vi "CreateDatabase.vi"(8 "错误输入（无错误）":errorcluster, 11 "测试类型":string) -> (0 "error out":errorcluster, 3 "数据库地址":string)   [LabVIEW 2014]
uses:
  <vilib>/addons/database/Connection.llb/DB Tools Open Connec (String).vi
  <vilib>/addons/database/Connection.llb/Conn Execute.vi
  <vilib>/addons/database/Recordset.llb/Rec Destroy - Connection.vi
  <vilib>/addons/database/NI_Database_API.lvlib
panel:
  out "error out 2":errorcluster
  out "连接的字符串 2":string
  in  "ADOX._Catalog":refnum<k7>
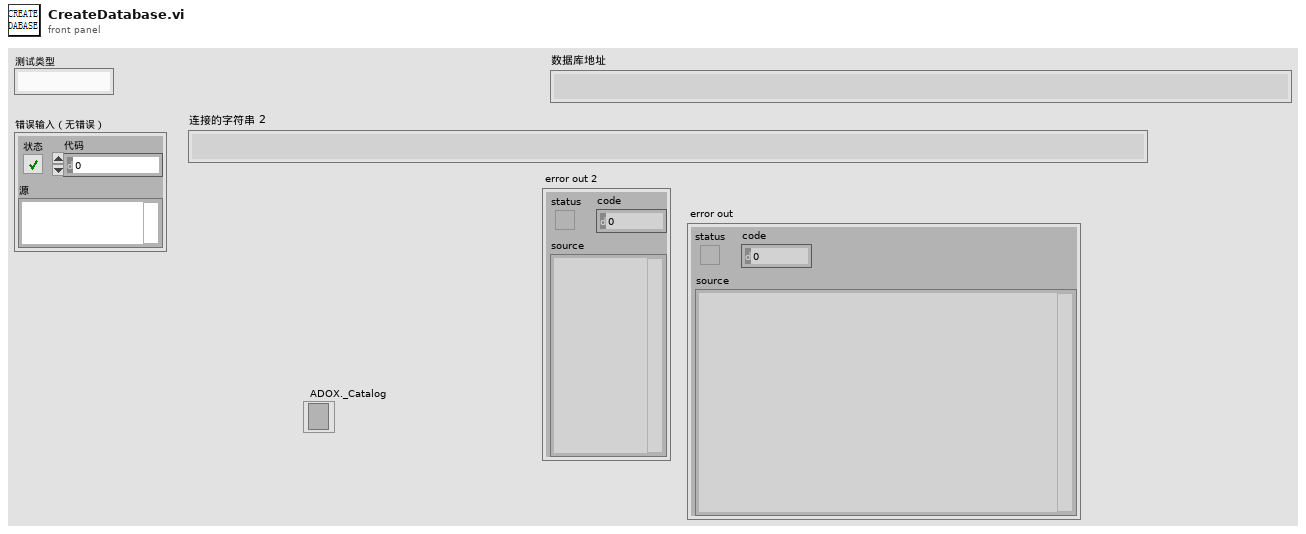
[diagram p1: front panel]
types:
  T1 = typedef "NI_Database_API.lvlib/Conn ObjectReference.ctl" = refnum<k1>
  T2 = typedef "NI_Database_API.lvlib/Rec ObjectReference.ctl" = refnum<k1>
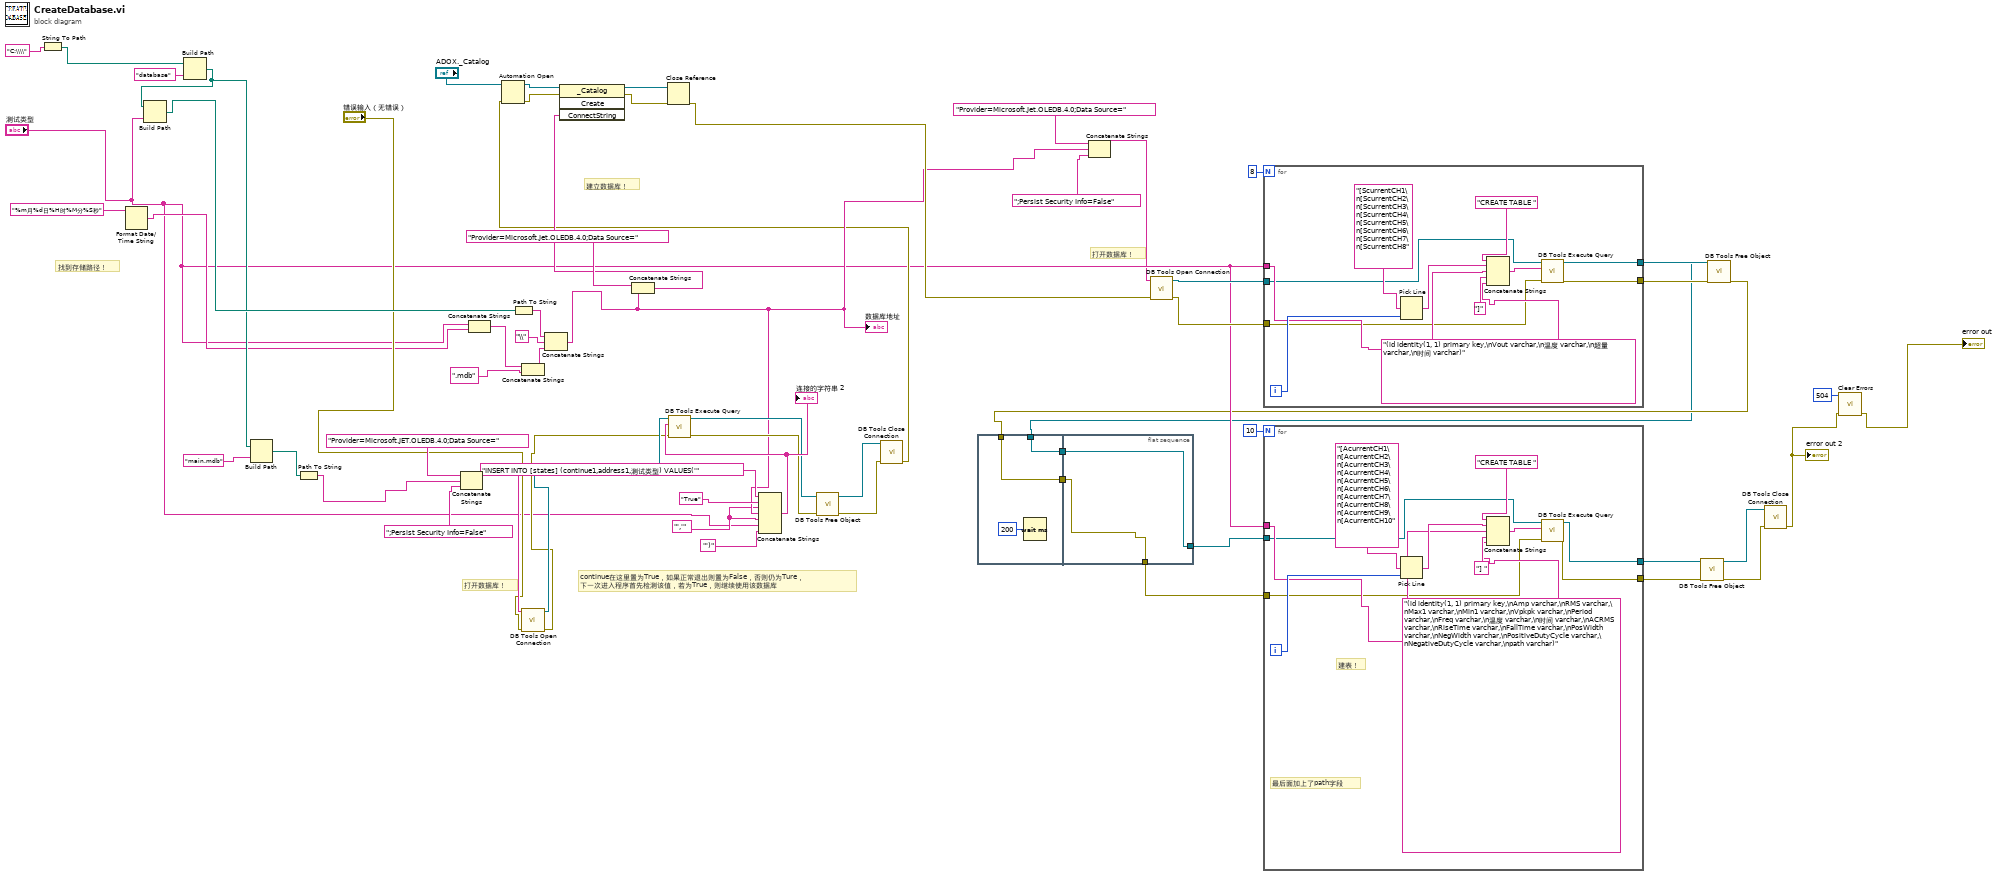
[diagram p0: block diagram]
diagram:
  w17 = "','"
  # "打开数据库！"
  # "continue在这里置为True，如果正常退出则置为False，否则仍为Ture，\n下一次进入程序首先检测该值，若为True，则继续使用该数据库"
  # "打开数据库！"
  # "建立数据库！"
  # "找到存储路径！"
  n1 = String To Path(string="C:\\\\") -> (path=w1:path)
  n2 = Format Date/Time String(time format string (%c)="%m月%d日%H时%M分%S秒" ("时间格式字符串(%c)")) -> (date/time string=w23:string)  [unwired: 2 in]
  n3 = Build Path(base path=w1, name or relative path="database" ("名称或相对路径")) -> (appended path=w34:path)
  n4 = Build Path(base path=w34, name or relative path="测试类型") -> (appended path=w49:path)
  n5 = Build Path(base path=w34, name or relative path="main.mdb" ("名称或相对路径")) -> (appended path=w32:path)
  n6 = Path To String(path=w32) -> (string=w31:string)
  n7 = Concatenate Strings("Provider=Microsoft.JET.OLEDB.4.0;Data Source=", w31, ";Persist Security Info=False") -> (w38:string)
  n8 = Concatenate Strings("测试类型", w23) -> (w20:string)
  n9 = Path To String(path=w49) -> (string=w51:string)
  n10 = Concatenate Strings(w20, ".mdb" ("字符串")) -> (w21:string)
  n11 = call-poly <vilib>:"DB Tools Open Connection.vi"("error in (no error)"="错误输入（无错误）", "connection information"=w38) -> ("error out"=w29:errorcluster, "connection reference"=w30:T1)  [unwired: 6 in]
  n12 = Concatenate Strings(w51, "\\" ("字符串"), w21) -> (w19:string)
  "数据库地址" <- w19
  n13 = Concatenate Strings("Provider=Microsoft.Jet.OLEDB.4.0;Data Source=", w19) -> (w57:string)
  n14 = Concatenate Strings("INSERT INTO [states] (continue1,address1,测试类型) VALUES('", "True", w17, w19, w17, "测试类型", "')") -> (w35:string)
  "连接的字符串 2" <- w35
  n15 = call-poly <vilib>:"DB Tools Execute Query.vi"("error in (no error)"=w29, "SQL query"=w35, "connection reference"=w30) -> ("error out"=w24:errorcluster, "recordset reference"=w25:T2)  [unwired: 5 in]
  n16 = call-poly <vilib>:"DB Tools Free Object.vi"("error in (no error)"=w24, "recordset reference"=w25) -> ("error out"=w26:errorcluster, "connection reference"=w27:T1)  [unwired: 8 in]
  n17 = call <vilib>:"DB Tools Close Connection.vi"("error in (no error)"=w26, "connection reference"=w27) -> ("error out"=w18:errorcluster)  [unwired: 5 in]
  n18 = Automation Open(error in (no error)=w18, Automation Refnum="ADOX._Catalog") -> (Automation Refnum=w62:refnum<k7>, error out=w61:errorcluster)  [unwired: 2 in]
  n19 = invoke class="_Catalog" method="Create"(reference=w62, error in=w61, "ConnectString"=w57) -> (reference out=w60:refnum<k7>, error out=w59:errorcluster)  [unwired: 1 in, 2 out]
  n20 = Close Reference(reference=w60, error in (no error)=w59) -> (error out=w54:errorcluster)
  n21 = flat-sequence {
    tunnel: w8 -> [w65]
    tunnel: [w65] -> w12
    tunnel: w7 -> [w64]
    tunnel: [w64] -> w6
    tunnel: w12 -> [w67]
    tunnel: [w68] -> w10
    tunnel: [w67] -> w9
    tunnel: w6 -> [w68]
    frame #0 {
      n22 = Wait (ms)(milliseconds to wait=u32 200 ("等待时间（毫秒）")) -> ()  [unwired: 1 out]
    }
    frame #1 {
    }
  }
  n23 = Concatenate Strings("Provider=Microsoft.Jet.OLEDB.4.0;Data Source=", w19, ";Persist Security Info=False") -> (w11:string)
  n24 = call-poly <vilib>:"DB Tools Open Connection.vi"("error in (no error)"=w54, "connection information"=w11) -> ("error out"=w41:errorcluster, "connection reference"=w42:T1)  [unwired: 6 in]
  n25 = for {
    N: 8 -> [_]
    tunnel: "测试类型" -> [w75]
    tunnel: w42 -> [w72]
    tunnel: w41 -> [w71]
    tunnel: [w70] -> w14
    tunnel: [w69] -> w13
    i -> [w77]
    # "建表！"
    n26 = Pick Line(multi-line string="[ScurrentCH1\n[ScurrentCH2\n[ScurrentCH3\n[ScurrentCH4\n[ScurrentCH5\n[ScurrentCH6\n[ScurrentCH7\n[ScurrentCH8" ("多行字符串"), line index=w77) -> (output string=w79:string)  [unwired: 1 in]
    n27 = Concatenate Strings("CREATE TABLE ", w79, w75, "]", "(id identity(1, 1) primary key,\nVout varchar,\n温度 varchar,\n超量 varchar,\n时间 varchar)") -> (w76:string)
    n28 = call-poly <vilib>:"DB Tools Execute Query.vi"("error in (no error)"=w71, "SQL query"=w76, "connection reference"=w72) -> ("error out"=w69:errorcluster, "recordset reference"=w70:T2)  [unwired: 5 in]
  }
  n29 = for {
    N: 10 -> [_]
    tunnel: [w83] -> w45
    tunnel: [w87] -> w44
    tunnel: "测试类型" -> [w86]
    tunnel: w10 -> [w82]
    tunnel: w9 -> [w81]
    i -> [w89]
    # "最后面加上了path字段"
    # "建表！"
    n30 = Pick Line(multi-line string="[AcurrentCH1\n[AcurrentCH2\n[AcurrentCH3\n[AcurrentCH4\n[AcurrentCH5\n[AcurrentCH6\n[AcurrentCH7\n[AcurrentCH8\n[AcurrentCH9\n[AcurrentCH10" ("多行字符串"), line index=w89) -> (output string=w91:string)  [unwired: 1 in]
    n31 = Concatenate Strings("CREATE TABLE ", w91, w86, "] ", "(id identity(1, 1) primary key,\nAmp varchar,\nRMS varchar,\nMax1 varchar,\nMin1 varchar,\nVpkpk varchar,\nPeriod varchar,\nFreq varchar,\n温度 varchar,\n时间 varchar,\nACRMS varchar,\nRiseTime varchar,\nFallTime varchar,\nPosWidth varchar,\nNegWidth varchar,\nPositiveDutyCycle varchar,\nNegativeDutyCycle varchar,\npath varchar)") -> (w88:string)
    n32 = call-poly <vilib>:"DB Tools Execute Query.vi"("error in (no error)"=w81, "SQL query"=w88, "connection reference"=w82) -> ("error out"=w87:errorcluster, "recordset reference"=w83:T2)  [unwired: 5 in]
  }
  n33 = call-poly <vilib>:"DB Tools Free Object.vi"("error in (no error)"=w44, "recordset reference"=w45) -> ("error out"=w47:errorcluster, "connection reference"=w46:T1)  [unwired: 8 in]
  n34 = call-poly <vilib>:"DB Tools Free Object.vi"("error in (no error)"=w13, "recordset reference"=w14) -> ("error out"=w8:errorcluster, "connection reference"=w7:T1)  [unwired: 8 in]
  n35 = call <vilib>:"DB Tools Close Connection.vi"("error in (no error)"=w47, "connection reference"=w46) -> ("error out"=w5:errorcluster)  [unwired: 5 in]
  "error out 2" <- w5
  n36 = call <vilib>:"Clear Errors.vi"("error in (no error)"=w5, "specific error code to clear (0: all)"=504) -> ("error out"=→"error out":errorcluster)  [unwired: 4 in, 1 out]
